vi "Reset.vi"(8 "error in (no error)":errorcluster, 10 "Set decimation":bool=TRUE, 11 "RP Instrument in":refnum<class "RP Instrument.lvclass">) -> (0 "error out":errorcluster, 3 "RP Instrument out":refnum<class "RP Instrument.lvclass">)   [LabVIEW 2019, in "RP Instrument.lvclass"]
uses:
  RP Instrument.lvclass
  RP Command.ctl
  RP Instrument.lvclass/RP Instrument.ctl
  RP Communicator/RP Communicator.lvclass
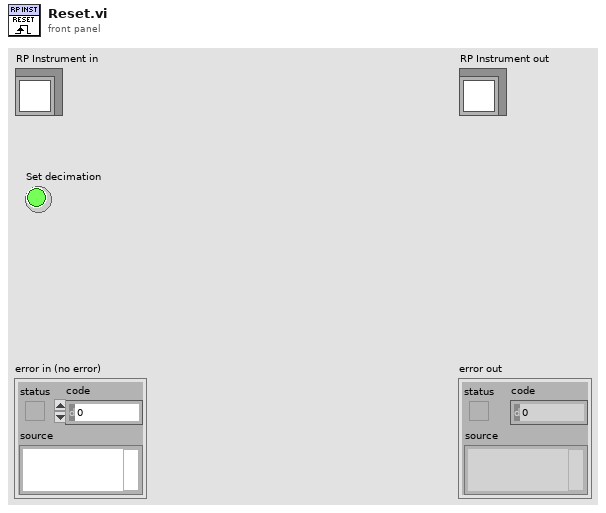
[diagram p1: front panel]
types:
  T1 = typedef "RP Command.ctl" = enum16{"Reset", "Read IDN", "Stop server", "Get status", "Get temperature", "Connect client", "Arm", "Software trigger", "Get whole buffer", "Get chunk", "System call", "Get config", "Set config", "Recieve data", "Recieve Calibartion", "Transmit data"}
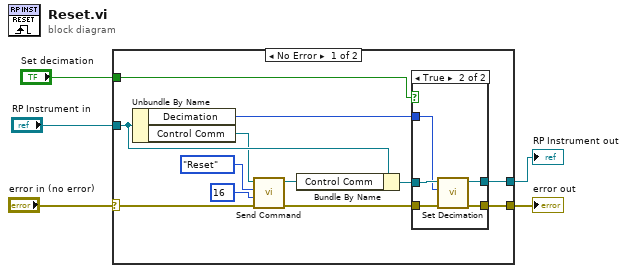
[diagram p0: block diagram]
diagram:
  n1 = case shown="No Error" "error in (no error)" {
    selector: "error in (no error)" -> [w12 w26]
    tunnel: [w10 w26] -> w4
    tunnel: [w8 w25] -> w2
    tunnel: "RP Instrument in" -> [w15 w25]
    tunnel: "Set decimation" -> [w7 _]
    frame No Error {
      n2 = Unbundle By Name(w15) -> ("Decimation"=w6:u32, "Control Comm"=w13:refnum<class "RP Communicator.lvclass">)
      n3 = call-dynamic "Send Command.vi"("error in (no error)"=w12, "Command payload"=u64 16, "Command number"=RP_Command."Reset", "RP Communicator in"=w13) -> ("error out"=w11:errorcluster, "RP Communicator out"=w14:refnum<class "RP Communicator.lvclass">)  [unwired: 6 in]
      n4 = Bundle By Name(cluster=w15, "Control Comm"=w14) -> (w9:refnum<class "RP Instrument.lvclass">)
      n5 = case shown="True" w7 {
        tunnel: w11 -> [w18 w24]
        tunnel: [w18 w23] -> w10
        tunnel: w9 -> [w19 w22]
        tunnel: [w19 w21] -> w8
        tunnel: w6 -> [_ w20]
        frame False {
        }
        frame True {
          n6 = call-dynamic "Set Decimation.vi"("error in (no error)"=w24, "Decimation"=w20, "RP Instrument in"=w22) -> ("error out"=w23:errorcluster, "RP Instrument out"=w21:refnum<class "RP Instrument.lvclass">)  [unwired: 7 in]
        }
      }
    }
    frame Error {
    }
  }
  "error out" <- w4
  "RP Instrument out" <- w2
